vi "MGCC_Commun_OutputChangedSetDigital (SubVI).vi"(11 "Array":T1[](array[typedef]) {"CROB value"."Control" items=["Nul"=0, "Pulse On"=1, "Pulse Off"=2, "Latch On"=3, "Latch Off"=4, "Close"=65, "Trip"=129]}) -> (1 "Numeric":i32, 3 "Array 2":T1[](array[typedef]) {"CROB value"."Control" items=["Nul"=0, "Pulse On"=1, "Pulse Off"=2, "Latch On"=3, "Latch Off"=4, "Close"=65, "Trip"=129]})   [LabVIEW 2016]
uses:
  <vilib>/DNP3/DNP3_Master/Crob With Index.ctl
  <vilib>/DNP3/DNP3_Common/crob.ctl
  <vilib>/DNP3/DNP3_Common/crob_ctrl.ctl
  <vilib>/DNP3/DNP3_Common.lvlib
  <vilib>/DNP3/DNP3_Master.lvlib
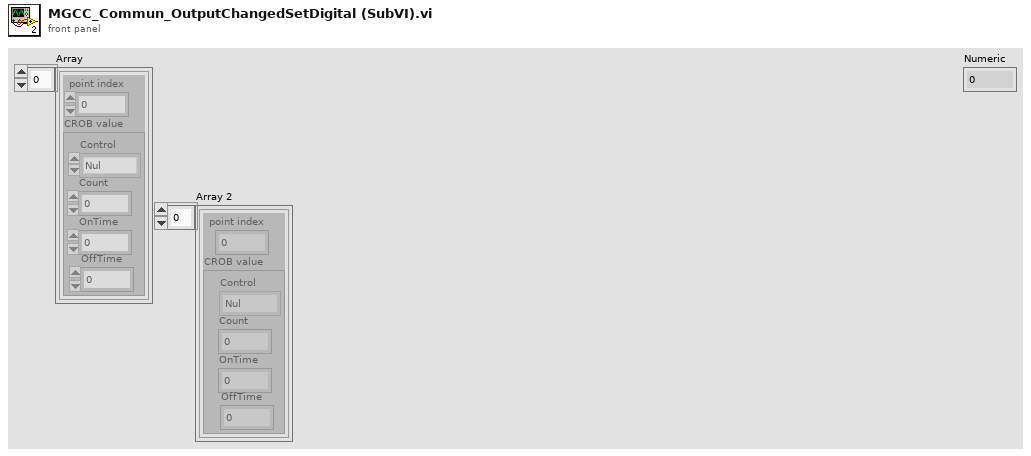
[diagram p1: front panel]
types:
  T1 = typedef "DNP3_Master.lvlib/Crob With Index.ctl" = cluster{"point index":u16, "CROB value":T2}
  T2 = typedef "DNP3_Common.lvlib/crob.ctl" = cluster{"OnTime":u32, "Count":u8, "OffTime":u32, "Control":T3}
  T3 = typedef "DNP3_Common.lvlib/crob_ctrl.ctl" = u8
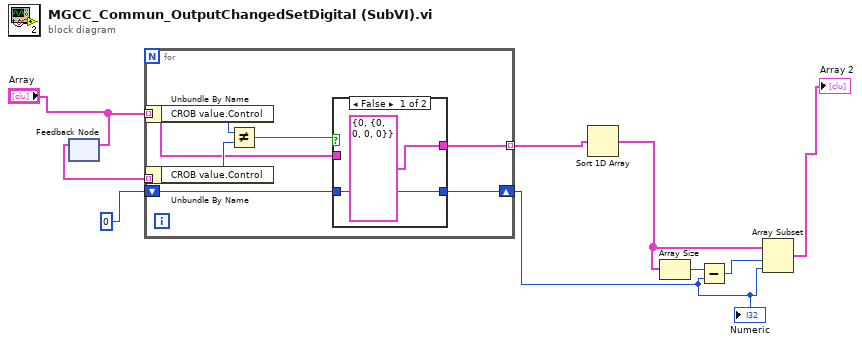
[diagram p0: block diagram]
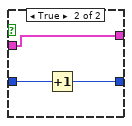
[diagram p2: hidden frame]
diagram:
  n1 = feedback #1() -> (w9:T1[])  [unwired: 1 in]
  n2 = feedback-in #1("Array") -> ()
  n3 = for {
    tunnel: "Array" -> [w10] mode=indexing
    tunnel: w9 -> [w17] mode=indexing
    shift-right: [w12] -> w3
    shift-left: 0 -> [w13]
    tunnel: [w11] -> w7 mode=indexing
    n4 = Unbundle By Name(w10) -> ("CROB value.Control"=w16:T3)
    n5 = Unbundle By Name(w17) -> ("CROB value.Control"=w15:T3)
    n6 = Not Equal?(x=w16, y=w15) -> (x != y?=w14:bool)
    n7 = case shown="False" w14 {
      tunnel: w13 -> [w19 w22]
      tunnel: [w19 w20] -> w12
      tunnel: [T1 {"point index"=0, "CROB value"={"OnTime"=0, "Count"=0, "OffTime"=0, "Control"=0}} ("CROB with point index") w21] -> w11
      tunnel: w10 -> [_ w21]
      frame False {
      }
      frame True {
        n8 = Increment(x=w22) -> (x+1=w20:i32)
      }
    }
  }
  "Numeric" <- w3
  n9 = Sort 1D Array(array=w7) -> (sorted array=w5:T1[])
  n10 = Array Size(array=w5) -> (size(s)=w6:i32)
  n11 = Subtract(x=w6, y=w3) -> (x-y=w4:i32)
  n12 = Array Subset(array=w5, index=w4, length=w3) -> (→"Array 2":T1[])
